vi "LV86_And.vi"(0 "Constant":u8=1, 2 "Image 2":T1={"Width"=0, "Height"=0, "Depth"=-1, "data"=[], "Compressed data"=[], "Color table"=[], "Duration"=0, "Options"=0, "Timestamp"=0, "ID"=0, "Reserved"=0, "Dialogs"=0} {"Dialogs" format="%.0b"}, 3 "Image":T1 {"Dialogs" format="%.0b"}) -> (1 "Image Out":T1 {"Dialogs" format="%.0b"})   [LabVIEW 2024]
doc: "This VI performs a boolean comparison between two binary images pixel by pixel or a constant to one image. If <B>Image 2</B> is unwired, the <B>constant</B> is compared to the image."
uses:
  <userlib>/ImageProcessing/QTLIB_2595_LV86/QT_Image.ctl
panel:
  # "This VI ANDs two images pixel by pixel or a constant\n to one image.  If Image 2 is unwired, the constant \nis ANDed to the image. (Does not work on a color image)"
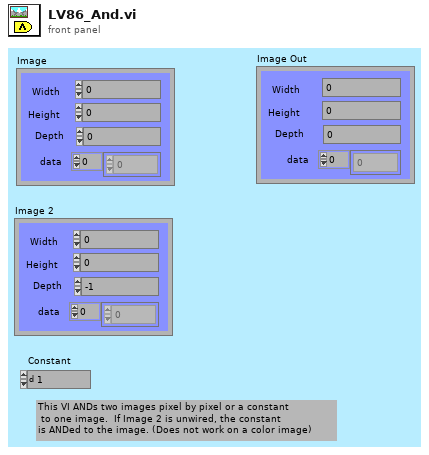
[diagram p1: front panel]
types:
  T1 = typedef "QT_Image.ctl" = cluster{"Width":i32, "Height":i32, "Depth":i32, "data":u8[], "Compressed data":u8[], "Color table":u32[], "Duration":i32, "Options":i32, "Timestamp":i32, "ID":i32, "Reserved":i32, "Dialogs":u32}
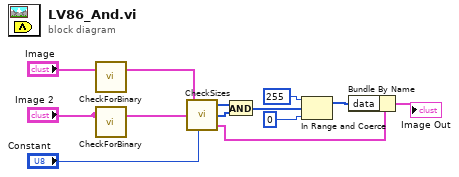
[diagram p0: block diagram]
diagram:
  n1 = call <userlib>:"CheckForBinary.vi"("Image in"="Image") -> ()  [unwired: 3 out]
  n2 = call <userlib>:"CheckForBinary.vi"("Image in"="Image 2") -> ()  [unwired: 3 out]
  n3 = call <userlib>:"CheckSizes.vi"("Constant"="Constant", "Image 2"="Image 2", "Image"="Image") -> ("Image template"=w5:T1, "Image 2 data"=w3:u8[], "Image 1 data"=w4:i32[])
  n4 = And(x=w4, y=w3) -> (x .and. y?=w8:i32[])
  n5 = In Range and Coerce(upper limit=u8 255, x=w8, lower limit=u8 0) -> (coerced(x)=w11:i32[])  [unwired: 1 out]
  n6 = Bundle By Name(cluster=w5, "data"=w11) -> (→"Image Out":T1)
